vi "uploadFile.vi"(8 "error in (no error)":errorcluster, 11 "uploadFileCluster":T1) -> (0 "error out":errorcluster)   [LabVIEW 2013, in "SlackinLabViewLib.lvlib"]
uses:
  <vilib>/httpClient/ClientHandle.ctl
  Controls/uploadFileCluster.ctl
  <vilib>/httpClient/MultipartData.ctl
  SlackinLabViewLib.lvlib
  <vilib>/httpClient/LabVIEWHTTPClient.lvlib
panel:
  out "client handle out":T2
  out "headers":string
  out "body":string
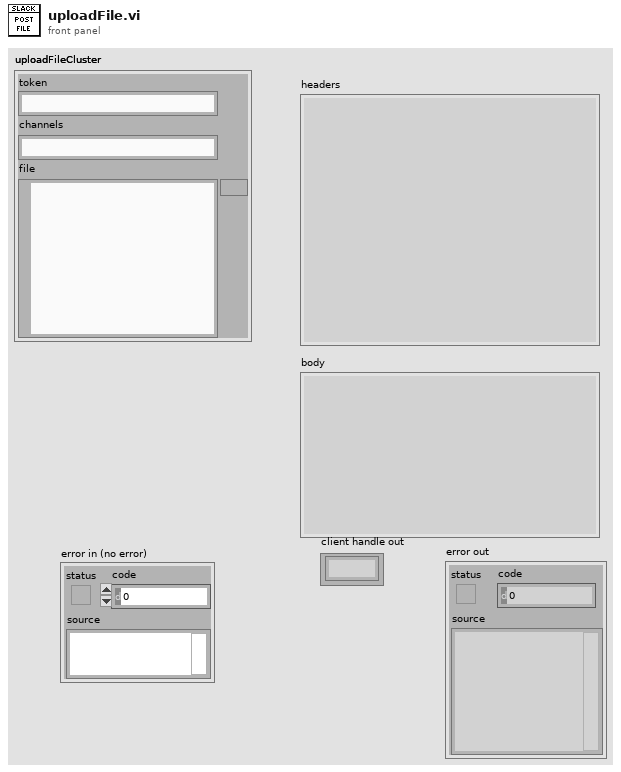
[diagram p1: front panel]
types:
  T1 = typedef "uploadFileCluster.ctl" = cluster{"token":string, "channels":string, "file":path}
  T2 = typedef "LabVIEWHTTPClient.lvlib/ClientHandle.ctl" = refnum<k1>
  T3 = typedef "LabVIEWHTTPClient.lvlib/MultipartData.ctl" = cluster{"Name":string, "Value":string, "File":path, "Filename":string, "MIME type":string}
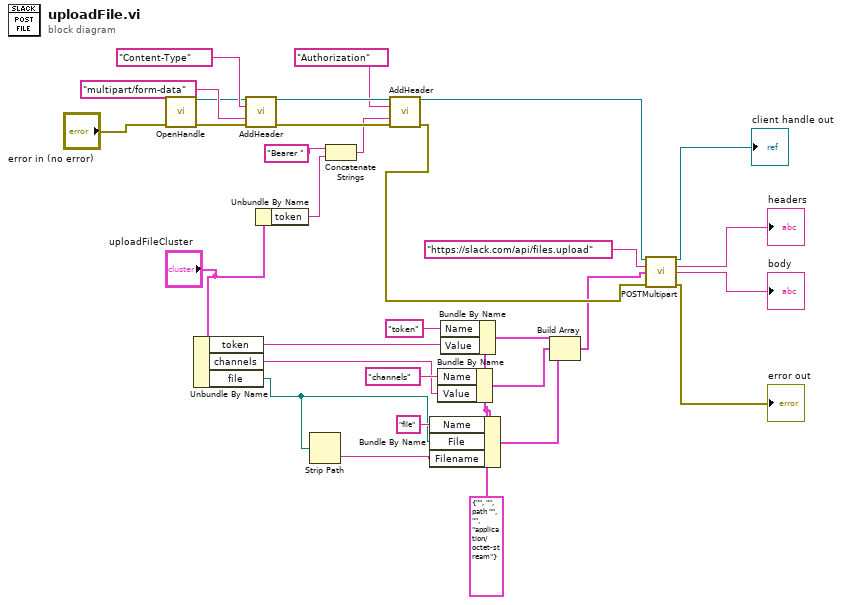
[diagram p0: block diagram]
diagram:
  w3 = T3 {"Name"="", "Value"="", "File"=path "", "Filename"="", "MIME type"="application/octet-stream"} ("Element")
  n1 = call <vilib>:"OpenHandle.vi"("error in (no error)"="error in (no error)") -> ("client handle out"=w24:T2, "error out"=w20:errorcluster)  [unwired: 13 in]
  n2 = Unbundle By Name("uploadFileCluster") -> ("token"=w10:string, "channels"=w6:string, "file"=w1:path)
  n3 = call <vilib>:"AddHeader.vi"("client handle"=w24, "header"="Content-Type", "value"="multipart/form-data", "error in (no error)"=w20) -> ("client handle out"=w22:T2, "error out"=w21:errorcluster)  [unwired: 10 in]
  n4 = Unbundle By Name("uploadFileCluster") -> ("token"=w16:string)
  n5 = Strip Path(path=w1) -> (name=w2:string)  [unwired: 1 out]
  n6 = Concatenate Strings("Bearer " ("string"), w16) -> (w18:string)
  n7 = call <vilib>:"AddHeader.vi"("client handle"=w22, "header"="Authorization", "value"=w18, "error in (no error)"=w21) -> ("client handle out"=w23:T2, "error out"=w14:errorcluster)  [unwired: 10 in]
  n8 = Bundle By Name(cluster=w3, "Name"="file", "File"=w1, "Filename"=w2) -> (w4:T3)
  n9 = Bundle By Name(cluster=w3, "Name"="channels", "Value"=w6) -> (w8:T3)
  n10 = Bundle By Name(cluster=w3, "Name"="token", "Value"=w10) -> (w9:T3)
  n11 = Build Array(w9, w8, w4) -> (w12:T3[])
  n12 = call <vilib>:"POSTMultipart.vi"("client handle"=w23, "url"="https://slack.com/api/files.upload", "data"=w12, "error in (no error)"=w14) -> ("client handle out"=→"client handle out":T2, "headers"=→"headers":string, "body"=→"body":string, "error out"=→"error out":errorcluster)  [unwired: 8 in]
